vi "ACT_Loop.vi"() -> ()   [LabVIEW 2023, in "Shooter_ACT.lvlib"]
uses:
  Shooter_ACT.lvlib
  Cluster_CMD_ACT_Data.ctl
  ENUM_Shooter_Mode.ctl
  Cluster_Shooter Status.ctl
  Cluster_Speed Sensor Values.ctl
  Cluster_Velocity Values.ctl
  Cluster_Voltage Values.ctl
  ENUM_ACT_State.ctl
  <vilib>/Rock Robotics/WPI/MotorControl/WPI_MotorControlDeviceRef.ctl
  <vilib>/Rock Robotics/WPI/MotorControl/WPI_MotorControlType.ctl
  <vilib>/Rock Robotics/SystemInterfaces/DIO/FPGA_DIOPWMChannel.ctl
  <vilib>/Rock Robotics/WPI/PWM/WPI_PWMDeadband.ctl
  <vilib>/Rock Robotics/SystemInterfaces/DIO/FPGA_DIOChannel.ctl
  <vilib>/Rock Robotics/WPI/ThirdParty/REV Robotics/REVLib/Typedef/Spark MAX Control Type.ctl
  ENUM_ACT_Action.ctl
  <vilib>/Rock Robotics/WPI/ThirdParty/REV Robotics/REVLib/Typedef/Spark MAX Idle Mode.ctl
  <vilib>/Rock Robotics/WPI/ThirdParty/Phoenix-LabVIEW/Motor Controller/Controls/CTRE_Phoenix_MotorControl_ControlMode.ctl
  RoboRIO Utilities/Global_STOP.vi
  Global_CMD_ACT_Data In.vi
  Global_ACT_Data Out.vi
panel:
  out "Motor Status":T1
  out "Target RPM":dbl
  out "Input DBL Data":T5
  out "Output DBL Data":dbl
  out "Cycle Time (S)":dbl format="%.3g"
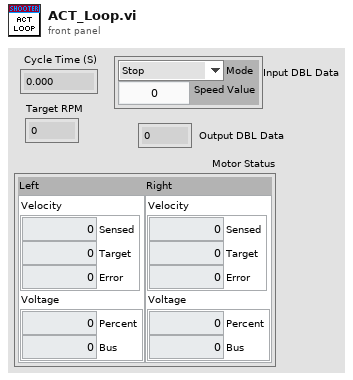
[diagram p1: front panel]
types:
  T1 = typedef "Shooter_ACT.lvlib/Cluster_Shooter Status.ctl" = cluster{"Left":T2, "Right":T2}
  T2 = typedef "Cluster_Speed Sensor Values.ctl" = cluster{"Velocity":T3, "Voltage":T4}
  T3 = typedef "Shooter_ACT.lvlib/Cluster_Velocity Values.ctl" = cluster{"Sensed":dbl, "Target":dbl, "Error":dbl}
  T4 = typedef "Shooter_ACT.lvlib/Cluster_Voltage Values.ctl" = cluster{"Percent":dbl, "Bus":dbl}
  T5 = typedef "Shooter_ACT.lvlib/Cluster_CMD_ACT_Data.ctl" = cluster{"Mode":T6, "Speed Value":dbl}
  T6 = typedef "Shooter_ACT.lvlib/ENUM_Shooter_Mode.ctl" = enum16{"Stop", "Speed Percent", "Speed RPM"}
  T7 = typedef "Spark MAX Control Type.ctl" = enum16{"Percent VBus", "Voltage", "Velocity", "Position", "Smart Motion", "Current", "Smart Velocity"}
  T8 = typedef "WPI_MotorControlDeviceRef.ctl" = cluster{"DeviceStatus":errorcluster, "Type":T9, "PWM":cluster{"PWM Channel":T10, "DeadBand":T11}, "CAN":cluster{"Device Number":u8, "SetOutput VI Ref":variant, "GetOutput VI Ref":variant, "Enable VI Ref":variant, "Disable VI Ref":variant, "Data":variant}, "Invert":bool, "DIO PWM":cluster{"PWM \"Enable\" Channel":T10, "DIOChannel":T12, "PWM Rate":dbl}}
  T9 = typedef "WPI_MotorControlType.ctl" = enum16{"PWM", "CAN", "DIO PWM"}
  T10 = typedef "FPGA_DIOPWMChannel.ctl" = enum8{"PWM 0", "PWM 1", "PWM 2", "PWM 3", "PWM 4", "PWM 5", "PWM 6", "PWM 7", "PWM 8", "PWM 9", "PWM MXP 0", "PWM MXP 1", "PWM MXP 2", "PWM MXP 3", "PWM MXP 4", "PWM MXP 5", "PWM MXP 6", "PWM MXP 7", "PWM MXP 8", "PWM MXP 9", "Invalid"}
  T11 = typedef "WPI_PWMDeadband.ctl" = cluster{"Name":string, "maxPositivePwm":i32, "minPositivePwm":i32, "centerPwm":i32, "maxNegativePwm":i32, "minNegativePwm":i32, "angularRange":u16}
  T12 = typedef "FPGA_DIOChannel.ctl" = enum8{"DIO 0", "DIO 1", "DIO 2", "DIO 3", "DIO 4", "DIO 5", "DIO 6", "DIO 7", "DIO 8", "DIO 9", "DIO MXP 0", "DIO MXP 1", "DIO MXP 2", "DIO MXP 3", "DIO MXP 4", "DIO MXP 5", "DIO MXP 6", "DIO MXP 7", "DIO MXP 8", "DIO MXP 9", "DIO MXP 10", "DIO MXP 11", "DIO MXP 12", "DIO MXP 13", "DIO MXP 14", "DIO MXP 15", "SPI Port CS1", "SPI Port CS2", "SPI Port CS3", "SPI Port MISO", "SPI Port MOSI", "Invalid"}
  T13 = typedef "Shooter_ACT.lvlib/ENUM_ACT_State.ctl" = enum16{"Starting", "Stopping", "Shooting", "Shutdown"}
  T14 = typedef "Shooter_ACT.lvlib/ENUM_ACT_Action.ctl" = enum16{"No Action", "Reset Time", "Reset All", "Setup Motors", "Setup Sensors", "Stop", "Set Speed RPM", "Set Speed Percent"}
  T15 = cluster{"Left Motor":T8, "Right Motor":T8, "State":T13, "Previous State":T13, "Current Time":timestamp, "Previous Time":timestamp, "Start Time":timestamp, "Target Time (ms)":u32, "Cycle Time(S)":dbl, "ACT Input":T5, "Motor Value":dbl, "Control Mode":T7, "Target RPM":dbl, "Motor Status":T1}
  T16 = typedef "Spark MAX Idle Mode.ctl" = enum16{"Coast", "Brake"}
  T17 = typedef "CTRE_Phoenix_MotorControl_ControlMode.ctl" = u16
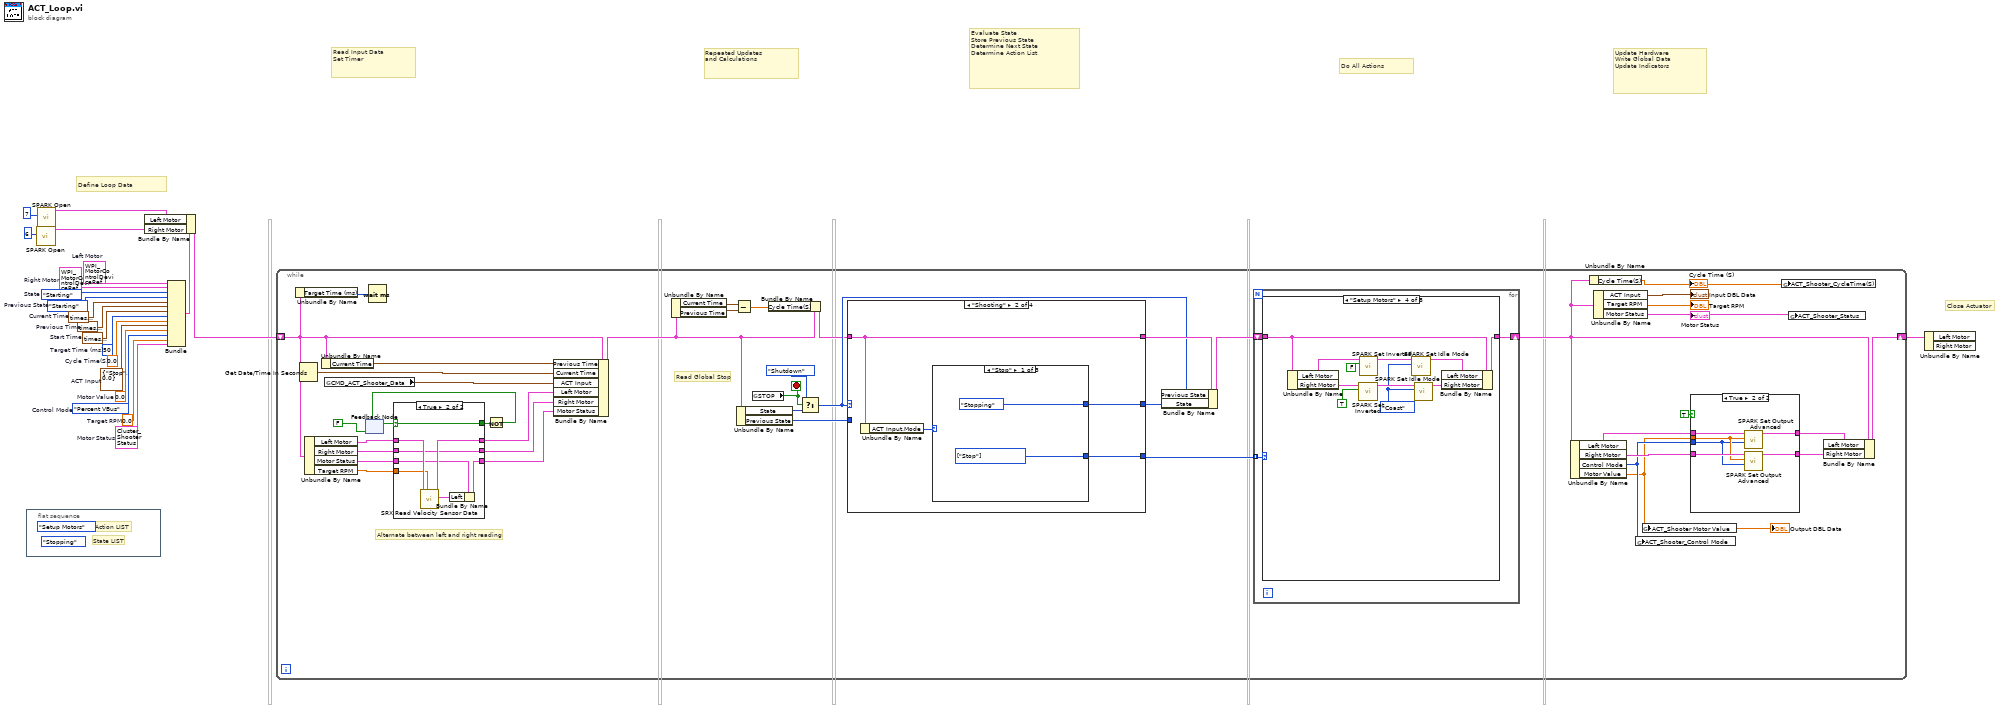
[diagram p0: block diagram]
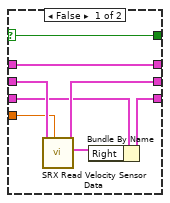
[diagram p3: hidden frame]
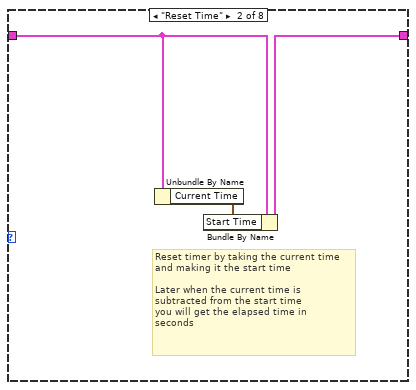
[diagram p5: hidden frame]
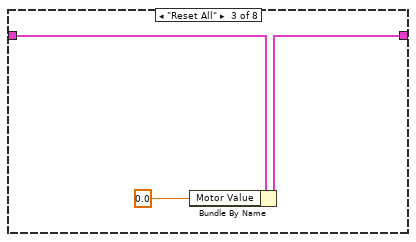
[diagram p6: hidden frame]
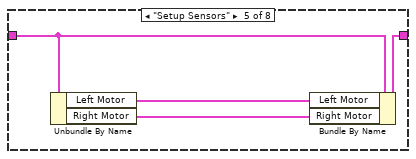
[diagram p7: hidden frame]
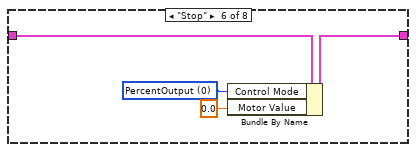
[diagram p8: hidden frame]
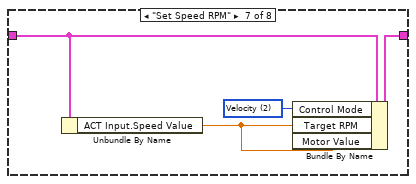
[diagram p9: hidden frame]
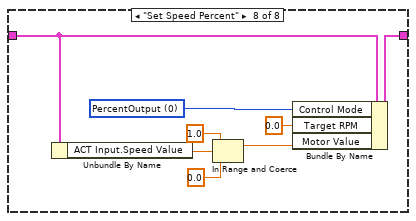
[diagram p10: hidden frame]
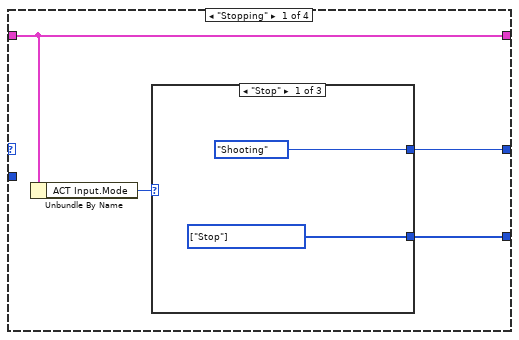
[diagram p11: hidden frame]
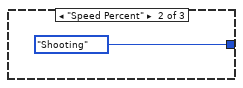
[diagram p12: hidden frame]
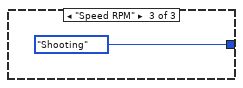
[diagram p13: hidden frame]
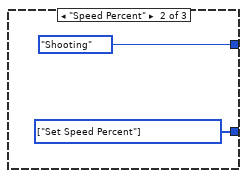
[diagram p14: hidden frame]
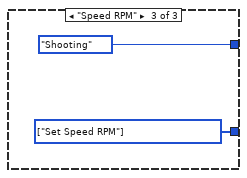
[diagram p15: hidden frame]
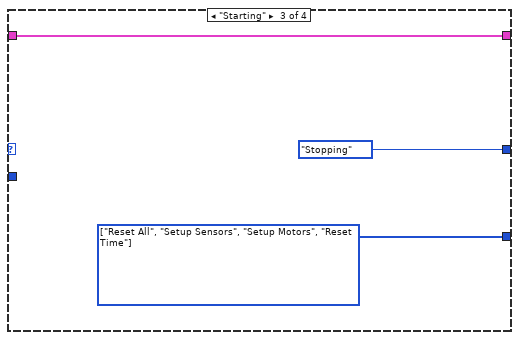
[diagram p16: hidden frame]
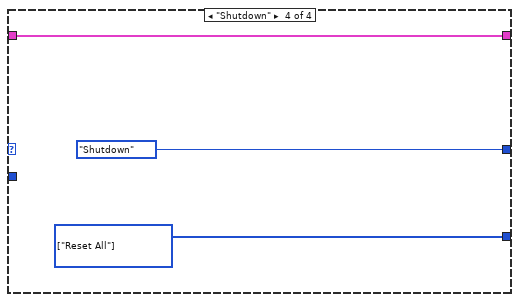
[diagram p17: hidden frame]
diagram:
  w1 = Spark_MAX_Control_Type."Percent VBus"  # Control Mode
  w6 = T1 {"Left"={"Velocity"={"Sensed"=0.0, "Target"=0.0, "Error"=0.0}, "Voltage"={"Percent"=0.0, "Bus"=0.0}}, "Right"={"Velocity"={"Sensed"=0.0, "Target"=0.0, "Error"=0.0}, "Voltage"={"Percent"=0.0, "Bus"=0.0}}}  # Motor Status
  w7 = 0.0  # Target RPM
  w9 = T8 {"DeviceStatus"={"status"=FALSE, "code"=0, "source"=""}, "Type"=enum."PWM", "PWM"={"PWM Channel"=enum."PWM 1", "DeadBand"={"Name"="", "maxPositivePwm"=0, "minPositivePwm"=0, "centerPwm"=0, "maxNegativePwm"=0, "minNegativePwm"=0, "angularRange"=0}}, "CAN"={"Device Number"=0, "SetOutput VI Ref"=variant(enum8{"Percent VBus", "Current", "Speed", "Position", "Voltage"} enum."Percent VBus"), "GetOutput VI Ref"=variant(refnum<k1> refnum), "Enable VI Ref"=variant(dbl 12.0), "Disable VI Ref"=variant(enum8{"Percent VBus", "Speed", "Position", "Slave", "Unchanged / Invalid", "Voltage Compensation", "Current", "Motion Profile"} enum."Percent VBus"), "Data"=variant}, "Invert"=FALSE, "DIO PWM"={"PWM \"Enable\" Channel"=enum."Invalid", "DIOChannel"=enum."Invalid", "PWM Rate"=0.0}}  # Right Motor
  w8 = T8 {"DeviceStatus"={"status"=FALSE, "code"=0, "source"=""}, "Type"=enum."PWM", "PWM"={"PWM Channel"=enum."PWM 1", "DeadBand"={"Name"="", "maxPositivePwm"=0, "minPositivePwm"=0, "centerPwm"=0, "maxNegativePwm"=0, "minNegativePwm"=0, "angularRange"=0}}, "CAN"={"Device Number"=0, "SetOutput VI Ref"=variant(enum8{"Percent VBus", "Current", "Speed", "Position", "Voltage"} enum."Percent VBus"), "GetOutput VI Ref"=variant(refnum<k1> refnum), "Enable VI Ref"=variant(dbl 12.0), "Disable VI Ref"=variant(enum8{"Percent VBus", "Speed", "Position", "Slave", "Unchanged / Invalid", "Voltage Compensation", "Current", "Motion Profile"} enum."Percent VBus"), "Data"=variant}, "Invert"=FALSE, "DIO PWM"={"PWM \"Enable\" Channel"=enum."Invalid", "DIOChannel"=enum."Invalid", "PWM Rate"=0.0}}  # Left Motor
  w13 = 0.0  # Cycle Time(S)
  w14 = ENUM_ACT_State."Starting"  # Previous State
  w15 = timestamp(0 s since 1904-01-01)  # Previous Time
  w16 = u32 50  # Target Time (ms)
  w17 = 0.0  # Motor Value
  w18 = T5 {"Mode"=enum."Stop", "Speed Value"=0.0}  # ACT Input
  w19 = timestamp(0 s since 1904-01-01)  # Start Time
  w20 = timestamp(0 s since 1904-01-01)  # Current Time
  w21 = ENUM_ACT_State."Starting"  # State
  # "Close Actuator"
  # "Define Loop Data"
  # "Repeated Updates\nand Calculations"
  # "Read Input Data\nSet Timer"
  # "Evaluate State\nStore Previous State\nDetermine Next State\nDetermine Action List"
  # "Do All Actions"
  # "Update Hardware\nWrite Global Data\nUpdate Indicators"
  n1 = flat-sequence {
    frame #0 {
      (unwired) ENUM_ACT_State."Stopping" ("State")
      (unwired) ENUM_ACT_Action."Setup Motors" ("Action")
      # "State LIST"
      # "Action LIST"
    }
  }
  n2 = call <vilib>:"SPARK Open.vi"("Device Number"=u8 6) -> ("MotorControlDeviceRef"=w5:T8)  [unwired: 9 in, 1 out]
  n3 = call <vilib>:"SPARK Open.vi"("Device Number"=u8 7) -> ("MotorControlDeviceRef"=w4:T8)  [unwired: 9 in, 1 out]
  n4 = Bundle("Left Motor"=w8, "Right Motor"=w9, "State"=w21, "Previous State"=w14, "Current Time"=w20, "Previous Time"=w15, "Start Time"=w19, "Target Time (ms)"=w16, "Cycle Time(S)"=w13, "ACT Input"=w18, "Motor Value"=w17, "Control Mode"=w1, "Target RPM"=w7, "Motor Status"=w6) -> (w11:T15)  [unwired: 1 in]
  n5 = Bundle By Name(cluster=w11, "Left Motor"=w4, "Right Motor"=w5) -> (w10:T15)
  n6 = while {
    shift-right: [w44] -> w12
    shift-left: w10 -> [w35]
    stop <- w60 stop-if-true
    # "Alternate between left and right reading"
    # "Read Global Stop"
    n7 = Unbundle By Name(w35) -> ("Target Time (ms)"=w57:u32)
    n8 = Get Date/Time In Seconds() -> (seconds since 1Jan1904=w64:timestamp)
    n9 = Unbundle By Name(w35) -> ("Left Motor"=w34:T8, "Right Motor"=w33:T8, "Motor Status"=w32:T1, "Target RPM"=w22:dbl)
    n10 = Unbundle By Name(w35) -> ("Current Time"=w56:timestamp)
    n11 = global read "Global_CMD_ACT_Data In.vi" "CMD_ACT_Shooter_Data"() -> (w46:T5)
    n12 = feedback #1(FALSE) -> (w26:bool)
    n13 = Wait (ms)(milliseconds to wait=w57) -> ()  [unwired: 1 out]
    n14 = case shown="True" w26 {
      selector: w26 -> [w74 w82]
      tunnel: w34 -> [w78 w88]
      tunnel: w33 -> [w80 w86]
      tunnel: w32 -> [w77 w84]
      tunnel: [w76 w85] -> w31
      tunnel: [w78 w87] -> w30
      tunnel: [w79 w86] -> w29
      tunnel: [w74 w82] -> w25
      tunnel: w22 -> [w73 w81]
      frame False {
        n15 = call "SRX Read Velocity Sensor Data.vi"("Target"=w73, "SRX Ref"=w80) -> ("Sensor Status Out"=w75:T2, "SRX Ref Out"=w79:T8)  [unwired: 7 in, 1 out]
        n16 = Bundle By Name(cluster=w77, "Right"=w75) -> (w76:T1)
      }
      frame True {
        n17 = call "SRX Read Velocity Sensor Data.vi"("Target"=w81, "SRX Ref"=w88) -> ("Sensor Status Out"=w83:T2, "SRX Ref Out"=w87:T8)  [unwired: 7 in, 1 out]
        n18 = Bundle By Name(cluster=w84, "Left"=w83) -> (w85:T1)
      }
    }
    n19 = Not(x=w25) -> (.not. x?=w24:bool)
    n20 = feedback-in #1(w24) -> ()
    n21 = Bundle By Name(cluster=w35, "Previous Time"=w56, "Current Time"=w64, "ACT Input"=w46, "Left Motor"=w30, "Right Motor"=w29, "Motor Status"=w31) -> (w51:T15)
    n22 = Unbundle By Name(w51) -> ("Current Time"=w52:timestamp, "Previous Time"=w53:timestamp)
    n23 = Subtract(x=w52, y=w53) -> (x-y=w49:dbl)
    n24 = Unbundle By Name(w51) -> ("State"=w58:T13, "Previous State"=w55:T13)
    n25 = global read "Global_STOP.vi" "STOP"() -> (w60:bool)
    n26 = Bundle By Name(cluster=w51, "Cycle Time(S)"=w49) -> (w50:T15)
    n27 = Select(t=ENUM_ACT_State."Shutdown" ("State"), s=w60, f=w58) -> (s? t:f=w54:T13)
    n28 = case shown="\"Shooting\"" w54 {
      tunnel: w50 -> [w131 w139 w150 w153]
      tunnel: [w131 w139 w150 w153] -> w62
      tunnel: [w132 w140 ENUM_ACT_State."Stopping" ("State") ENUM_ACT_State."Shutdown" ("State")] -> w61
      tunnel: [w133 w141 w148 w151] -> w48
      tunnel: w55 -> [_ _ _ _]
      frame "Stopping" {
        n29 = Unbundle By Name(w131) -> ("ACT Input.Mode"=w130:T6)
        n30 = case shown="\"Stop\"" w130 {
          tunnel: [w135 _ _] -> w133
          tunnel: [ENUM_ACT_State."Shooting" ("State") ENUM_ACT_State."Shooting" ("State") ENUM_ACT_State."Shooting" ("State")] -> w132
          frame "Stop" {
            w135 = T14[] [enum."Stop"] items=["No Action", "Reset Time", "Reset All", "Setup Motors", "Setup Sensors", "Stop", "Set Speed RPM", "Set Speed Percent"] ("Actions")
          }
          frame "Speed Percent" {
          }
          frame "Speed RPM" {
          }
        }
      }
      frame "Shooting" {
        n31 = Unbundle By Name(w139) -> ("ACT Input.Mode"=w138:T6)
        n32 = case shown="\"Stop\"" w138 {
          tunnel: [w142 w144 w146] -> w141
          tunnel: [ENUM_ACT_State."Stopping" ("State") ENUM_ACT_State."Shooting" ("State") ENUM_ACT_State."Shooting" ("State")] -> w140
          frame "Stop" {
            w142 = T14[] [enum."Stop"] items=["No Action", "Reset Time", "Reset All", "Setup Motors", "Setup Sensors", "Stop", "Set Speed RPM", "Set Speed Percent"] ("Actions")
          }
          frame "Speed Percent" {
            w144 = T14[] [enum."Set Speed Percent"] items=["No Action", "Reset Time", "Reset All", "Setup Motors", "Setup Sensors", "Stop", "Set Speed RPM", "Set Speed Percent"] ("Actions")
          }
          frame "Speed RPM" {
            w146 = T14[] [enum."Set Speed RPM"] items=["No Action", "Reset Time", "Reset All", "Setup Motors", "Setup Sensors", "Stop", "Set Speed RPM", "Set Speed Percent"] ("Actions")
          }
        }
      }
      frame "Starting" {
        w148 = T14[] [enum."Reset All", enum."Setup Sensors", enum."Setup Motors", enum."Reset Time"] items=["No Action", "Reset Time", "Reset All", "Setup Motors", "Setup Sensors", "Stop", "Set Speed RPM", "Set Speed Percent"] ("Actions")
      }
      frame "Shutdown" {
        w151 = T14[] [enum."Reset All"] items=["No Action", "Reset Time", "Reset All", "Setup Motors", "Setup Sensors", "Stop", "Set Speed RPM", "Set Speed Percent"] ("Actions")
      }
    }
    n33 = Bundle By Name(cluster=w62, "Previous State"=w54, "State"=w61) -> (w63:T15)
    n34 = for {
      tunnel: w48 -> [w91] mode=indexing
      shift-right: [w90] -> w45
      shift-left: w63 -> [w89]
      n35 = case shown="\"Setup Motors\"" w91 {
        tunnel: w89 -> [w92 w95 w98 w109 w113 w116 w119 w127]
        tunnel: [w92 w94 w97 w108 w112 w117 w121 w129] -> w90
        frame "No Action" {
        }
        frame "Reset Time" {
          # "Reset timer by taking the current time\nand making it the start time\n\nLater when the current time is \nsubtracted from the start time\nyou will get the elapsed time in \nseconds"
          n36 = Unbundle By Name(w95) -> ("Current Time"=w93:timestamp)
          n37 = Bundle By Name(cluster=w95, "Start Time"=w93) -> (w94:T15)
        }
        frame "Reset All" {
          n38 = Bundle By Name(cluster=w98, "Motor Value"=0.0 ("FG Write Value")) -> (w97:T15)
        }
        frame "Setup Motors" {
          w99 = Spark_MAX_Idle_Mode."Coast" ("Idle Mode")
          n39 = Unbundle By Name(w109) -> ("Left Motor"=w107:T8, "Right Motor"=w105:T8)
          n40 = call <vilib>:"SPARK Set Inverted.vi"("Inverted (F)"=TRUE ("Invert Right"), "MotorControlDeviceRef in"=w105) -> ("MotorControlDeviceRef out"=w100:T8)  [unwired: 8 in, 1 out]
          n41 = call <vilib>:"SPARK Set Inverted.vi"("Inverted (F)"=FALSE ("Invert Left"), "MotorControlDeviceRef in"=w107) -> ("MotorControlDeviceRef out"=w103:T8)  [unwired: 8 in, 1 out]
          n42 = call <vilib>:"SPARK Set Idle Mode.vi"("Idle Mode"=w99, "MotorControlDeviceRef in"=w103) -> ("MotorControlDeviceRef out"=w102:T8)  [unwired: 8 in, 1 out]
          n43 = call <vilib>:"SPARK Set Idle Mode.vi"("Idle Mode"=w99, "MotorControlDeviceRef in"=w100) -> ("MotorControlDeviceRef out"=w101:T8)  [unwired: 8 in, 1 out]
          n44 = Bundle By Name(cluster=w109, "Left Motor"=w102, "Right Motor"=w101) -> (w108:T15)
        }
        frame "Setup Sensors" {
          n45 = Unbundle By Name(w113) -> ("Left Motor"=w110:T8, "Right Motor"=w111:T8)
          n46 = Bundle By Name(cluster=w113, "Left Motor"=w110, "Right Motor"=w111) -> (w112:T15)
        }
        frame "Stop" {
          w115 = T17 0 items=["PercentOutput"=0, "Position"=1, "Velocity"=2, "Current"=3, "Follower"=5, "MotionProfile"=6, "MotionMagic"=7, "MotionProfileArc"=10, "Disabled"=15] ("Control Mode")
          n47 = Bundle By Name(cluster=w116, "Control Mode"=w115, "Motor Value"=0.0) -> (w117:T15)
        }
        frame "Set Speed RPM" {
          w120 = T17 2 items=["PercentOutput"=0, "Position"=1, "Velocity"=2, "Current"=3, "Follower"=5, "MotionProfile"=6, "MotionMagic"=7, "MotionProfileArc"=10, "Disabled"=15] ("Control Mode")
          n48 = Unbundle By Name(w119) -> ("ACT Input.Speed Value"=w118:dbl)
          n49 = Bundle By Name(cluster=w119, "Control Mode"=w120, "Target RPM"=w118, "Motor Value"=w118) -> (w121:T15)
        }
        frame "Set Speed Percent" {
          w128 = T17 0 items=["PercentOutput"=0, "Position"=1, "Velocity"=2, "Current"=3, "Follower"=5, "MotionProfile"=6, "MotionMagic"=7, "MotionProfileArc"=10, "Disabled"=15] ("Control Mode")
          n50 = Unbundle By Name(w127) -> ("ACT Input.Speed Value"=w125:dbl)
          n51 = In Range and Coerce(upper limit=1.0, x=w125, lower limit=0.0 ("upper limit")) -> (coerced(x)=w122:dbl)  [unwired: 1 out]
          n52 = Bundle By Name(cluster=w127, "Control Mode"=w128, "Target RPM"=0.0, "Motor Value"=w122) -> (w129:T15)
        }
      }
    }
    n53 = Unbundle By Name(w45) -> ("Left Motor"=w42:T8, "Right Motor"=w40:T8, "Control Mode"=w38:T7, "Motor Value"=w37:dbl)
    "Output DBL Data" <- w37
    n54 = Unbundle By Name(w45) -> ("Cycle Time(S)"=w43:dbl)
    "Cycle Time (S)" <- w43
    n55 = Unbundle By Name(w45) -> ("ACT Input"=→"Input DBL Data":T5, "Target RPM"=→"Target RPM":dbl, "Motor Status"=w28:T1)
    "Motor Status" <- w28
    n56 = global write "Global_ACT_Data Out.vi" "ACT_Shooter_Control Mode"(w38) -> ()
    n57 = global write "Global_ACT_Data Out.vi" "ACT_Shooter Motor Value"(w37) -> ()
    n58 = case shown="True" TRUE {
      tunnel: w42 -> [w66 w72]
      tunnel: [w66 w71] -> w41
      tunnel: w40 -> [w65 w70]
      tunnel: [w65 w69] -> w39
      tunnel: w38 -> [_ w67]
      tunnel: w37 -> [_ w68]
      frame False {
      }
      frame True {
        n59 = call <vilib>:"SPARK Set Output Advanced.vi"("Control Mode"=w67, "Setpoint"=w68, "MotorControlDevRef"=w72) -> ("MotorControlDevRef"=w71:T8)  [unwired: 7 in, 1 out]
        n60 = call <vilib>:"SPARK Set Output Advanced.vi"("Control Mode"=w67, "Setpoint"=w68, "MotorControlDevRef"=w70) -> ("MotorControlDevRef"=w69:T8)  [unwired: 7 in, 1 out]
      }
    }
    n61 = global write "Global_ACT_Data Out.vi" "ACT_Shooter_CycleTime(S)"(w43) -> ()
    n62 = global write "Global_ACT_Data Out.vi" "ACT_Shooter_Status"(w28) -> ()
    n63 = Bundle By Name(cluster=w45, "Left Motor"=w41, "Right Motor"=w39) -> (w44:T15)
  }
  n64 = Unbundle By Name(w12) -> ()  [unwired: 2 out]
